vi "Mexa parseWIN.vi"(10 "Byte array":u8[](array[numeric])=[6, 64, 24, 31, 2, 255, 167, 0, 3, 255, 54, 0, 0, 3, 231, 39, 15, 3, 234, 0, 21, 0, 0, 0, 0, 0, 0, 129]) -> (2 "Output":dbl[](array[numeric]))   [LabVIEW 2011]
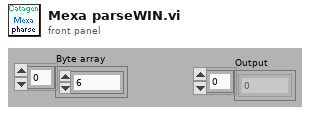
[diagram p1: front panel]
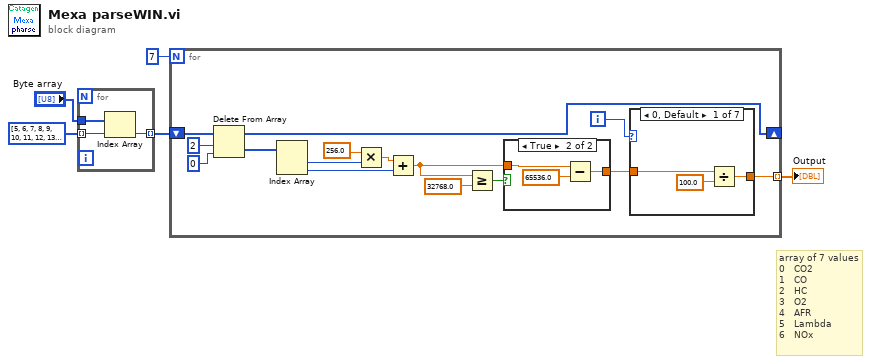
[diagram p0: block diagram]
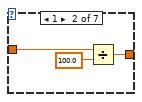
[diagram p2: hidden frame]
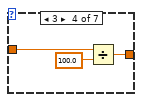
[diagram p4: hidden frame]
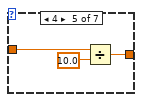
[diagram p5: hidden frame]
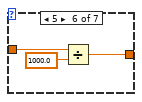
[diagram p6: hidden frame]
diagram:
  # "array of 7 values\n0   CO2\n1   CO\n2   HC\n3   O2\n4   AFR\n5   Lambda\n6   NOx"
  n1 = for {
    tunnel: "Byte array" -> [w8]
    tunnel: i32[] [5, 6, 7, 8, 9, 10, 11, 12, 13, 14, 15, 16, 21, 22] -> [w7] mode=indexing
    tunnel: [w6] -> w3 mode=indexing
    n2 = Index Array(array=w8, index=w7) -> (element=w6:u8)
  }
  n3 = for {
    N: 7 -> [_]
    tunnel: [w17] -> w1 mode=indexing
    shift-right: [w9] -> _
    shift-left: w3 -> [w13]
    i -> [w16]
    n4 = Delete From Array(array=w13, length=2, index=0 ("length")) -> (deleted portion=w12:u8[], array with subset deleted=w9:u8[])
    n5 = Index Array(array=w12) -> (element #1=w15:u8, element #2=w14:u8)  [unwired: 2 in]
    n6 = Multiply(x=256.0, y=w15) -> (x*y=w22:dbl)
    n7 = Add(x=w22, y=w14) -> (x+y=w19:dbl)
    n8 = Greater Or Equal?(x=w19, y=32768.0) -> (x >= y?=w21:bool)
    n9 = case shown="True" w21 {
      tunnel: w19 -> [w41 w44]
      tunnel: [w41 w43] -> w18
      frame False {
      }
      frame True {
        n10 = Subtract(x=w44, y=65536.0) -> (x-y=w43:dbl)
      }
    }
    n11 = case shown="0, Default" w16 {
      tunnel: w18 -> [w26 w27 w30 w31 w34 w37 w40]
      tunnel: [w24 w28 w30 w32 w35 w38 w40] -> w17
      frame 0, Default {
        n12 = Divide(x=w26, y=100.0) -> (x/y=w24:dbl)
      }
      frame 1 {
        n13 = Divide(x=w27, y=100.0) -> (x/y=w28:dbl)
      }
      frame 2 {
      }
      frame 3 {
        n14 = Divide(x=w31, y=100.0) -> (x/y=w32:dbl)
      }
      frame 4 {
        n15 = Divide(x=w34, y=10.0) -> (x/y=w35:dbl)
      }
      frame 5 {
        n16 = Divide(x=w37, y=1000.0) -> (x/y=w38:dbl)
      }
      frame 6 {
      }
    }
  }
  "Output" <- w1
